vi "Camera.vi"(8 "error in (no error)":errorcluster, 10 "Notifiers":T1, 11 "All Message Queue Cluster":T2) -> (0 "error out":errorcluster)   [LabVIEW 2013]
doc: "Ce VI est la partie visualisation du Spectrometre. Elle permet l'envoie d'ordre à cette appareil et affiche son état.\n- Connected : indique si l'appareil est connecté.\n- Acquiring : indique si le spectrometre acquière.\n- Status : indique le status actuel du spectromètre. CAD s'il y a une erreur, ou s'il est en mouvement, etc ..."
uses:
  Lib QMH/AllMessageQueue Cluster.ctl
  Lib QMH/Message Cluster.ctl
  Lib Notifier/Notifier.ctl
  Camera UI data.ctl
  <vilib>/vision/Image Controls.llb/IMAQ Image.ctl
  Camera config.ctl
  Lib IHM Control/Front Panel Status.ctl
  support/Status.vi
  Lib QMH/MessageQueues.lvlib
  Lib IHM Control/IHM Control.lvlib
  Lib Notifier/Notifier.lvlib
panel:
  out "Acquiring":bool
  out "Status":string
  out "Connected":bool
  # "Camera"
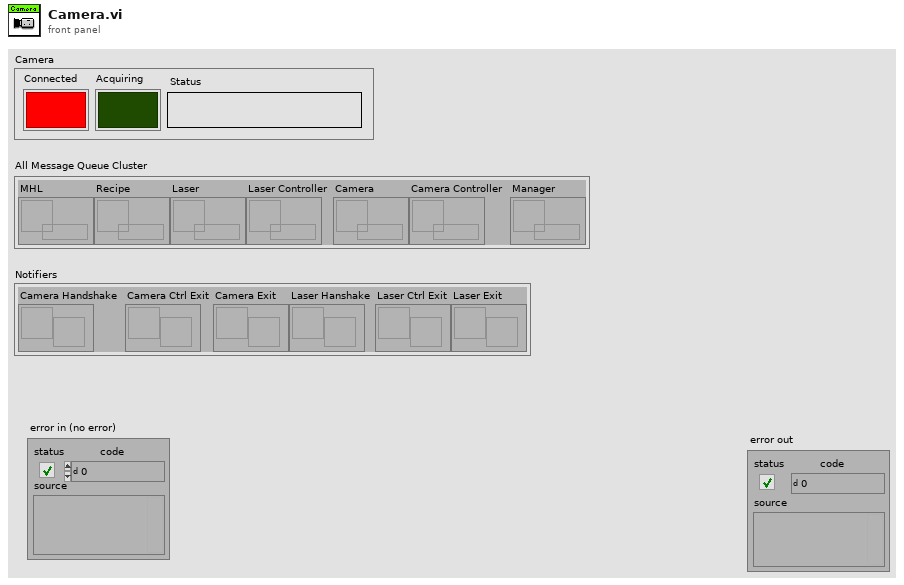
[diagram p1: front panel]
types:
  T1 = typedef "Notifier.lvlib/Notifier.ctl" = cluster{"Camera Handshake":refnum<notifier>, "Camera Ctrl Exit":refnum<notifier>, "Camera Exit":refnum<notifier>, "Laser Hanshake":refnum<notifier>, "Laser Ctrl Exit":refnum<notifier>, "Laser Exit":refnum<notifier>}
  T2 = typedef "MessageQueues.lvlib/AllMessageQueue Cluster.ctl" = cluster{"MHL":refnum<queue>, "Recipe":refnum<queue>, "Laser":refnum<queue>, "Laser Controller":refnum<queue>, "Camera":refnum<queue>, "Camera Controller":refnum<queue>, "Manager":refnum<queue>}
  T3 = typedef "IHM Control.lvlib/Front Panel Status.ctl" = enum16{"Initialisation", "Enable Laser", "Enable Camera", "Disable Laser", "Disable Camera"}
  T4 = typedef "Image Type" = u32
  T5 = typedef "Camera config.ctl" = cluster{"VISA resource name":refnum<visa-resource-name>}
  T6 = typedef "Camera UI data.ctl" = cluster{"Connected":bool, "Status":string, "Acquiring":bool, "Image":T7}
  T7 = typedef "IMAQ Image.ctl" = refnum<image>
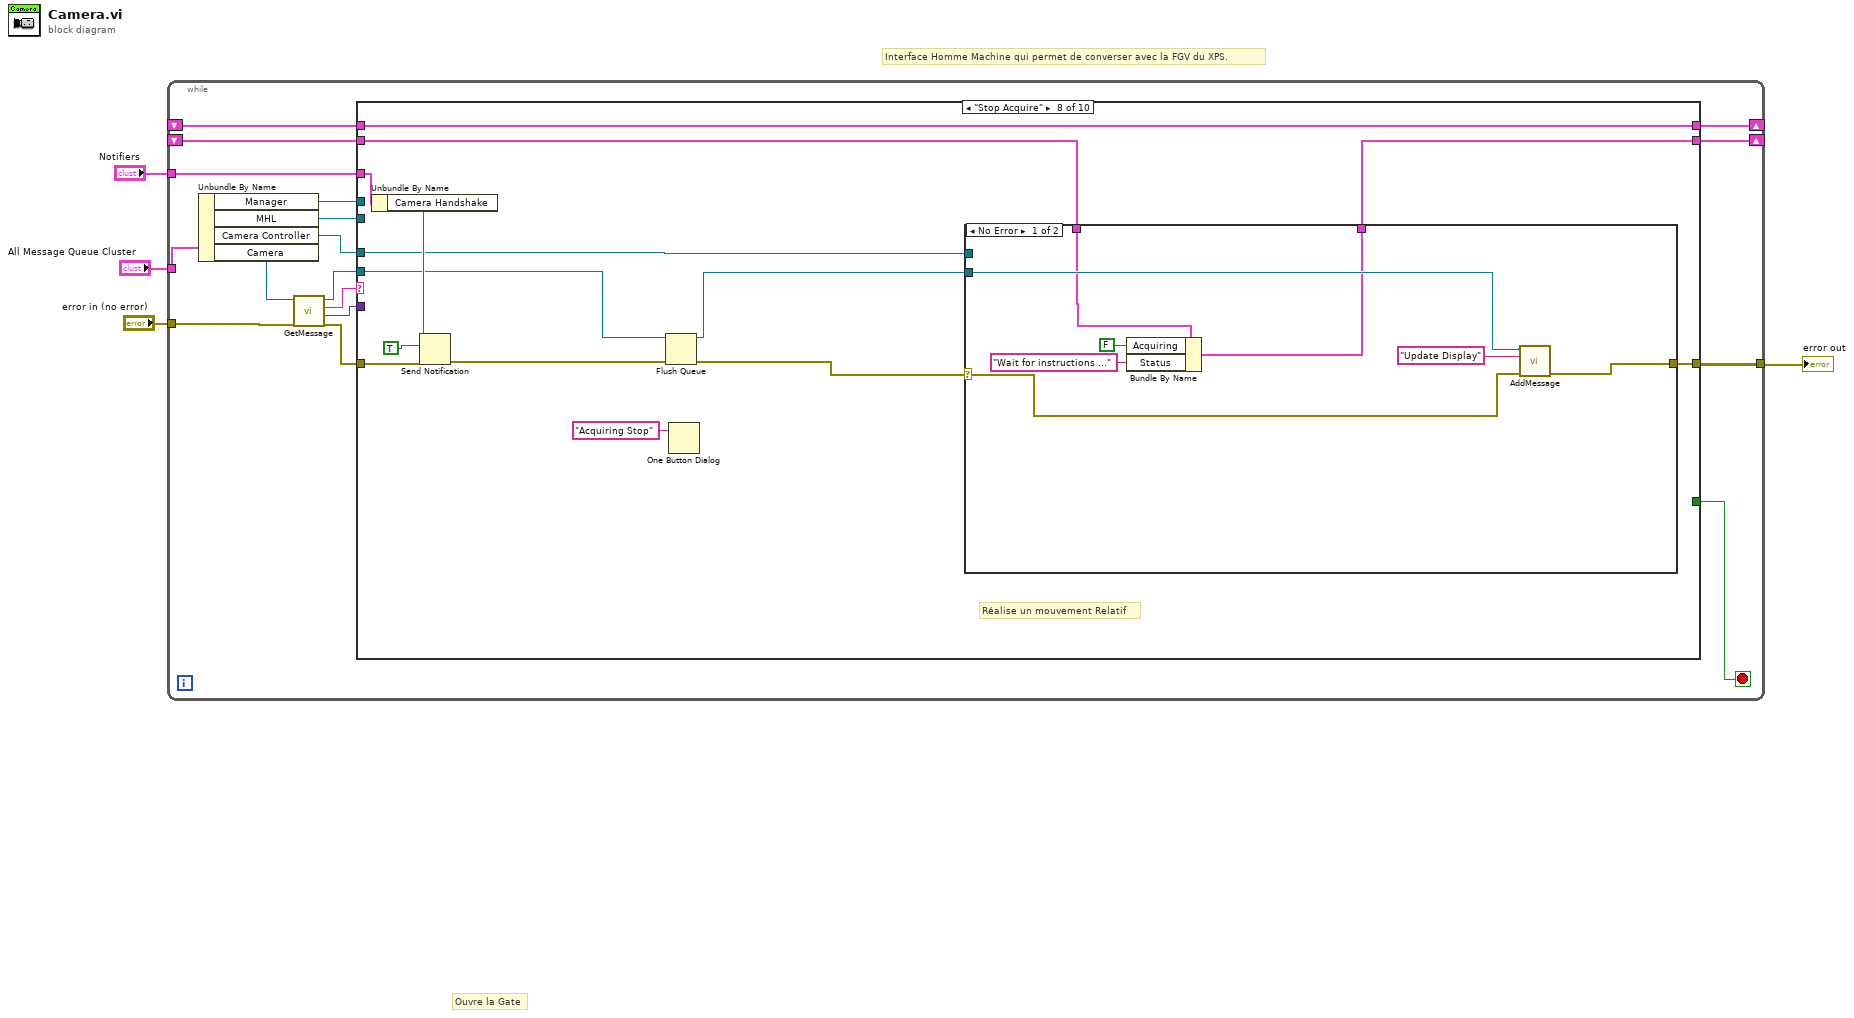
[diagram p0: block diagram]
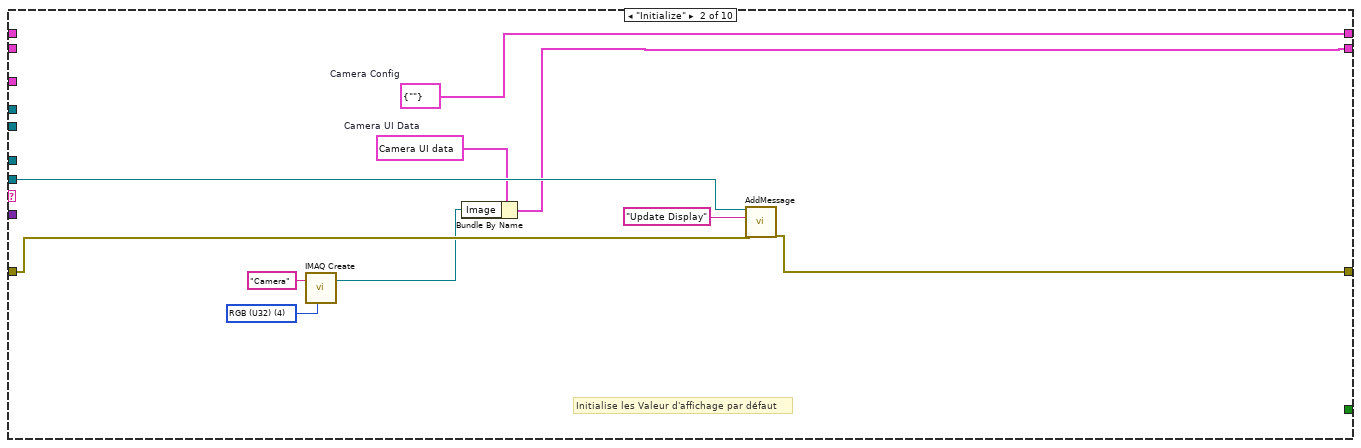
[diagram p3: hidden frame]
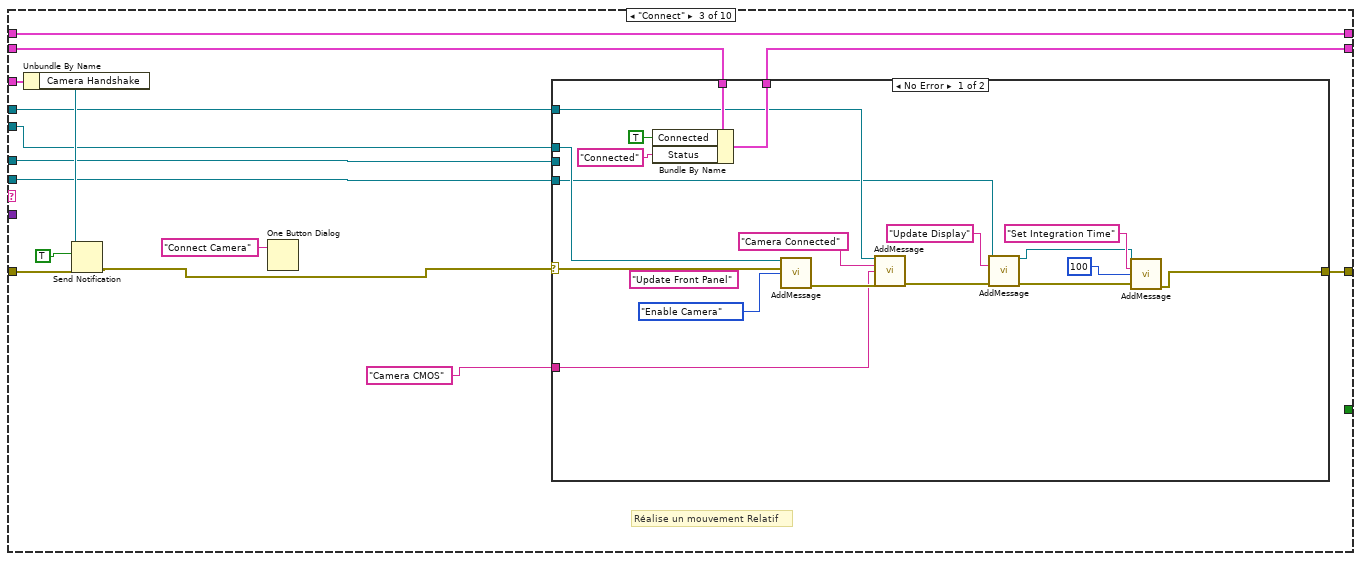
[diagram p4: hidden frame]
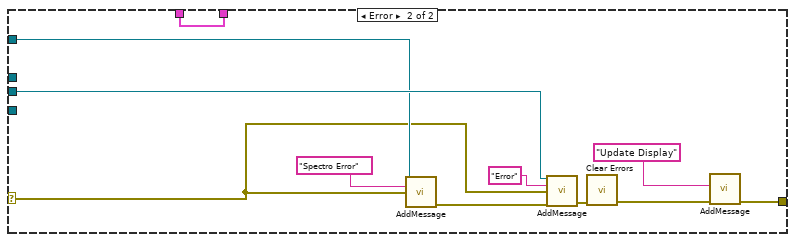
[diagram p5: hidden frame]
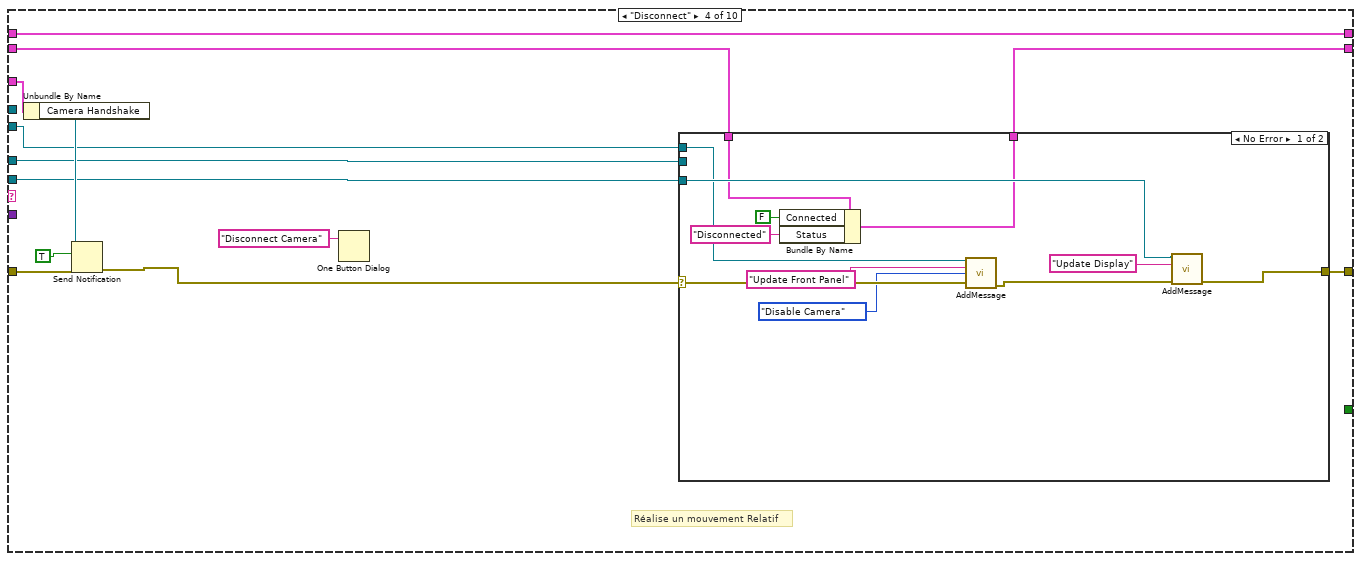
[diagram p6: hidden frame]
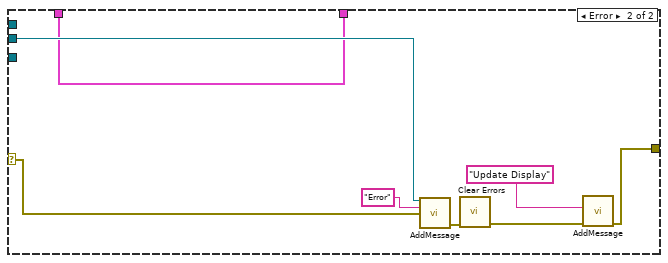
[diagram p7: hidden frame]
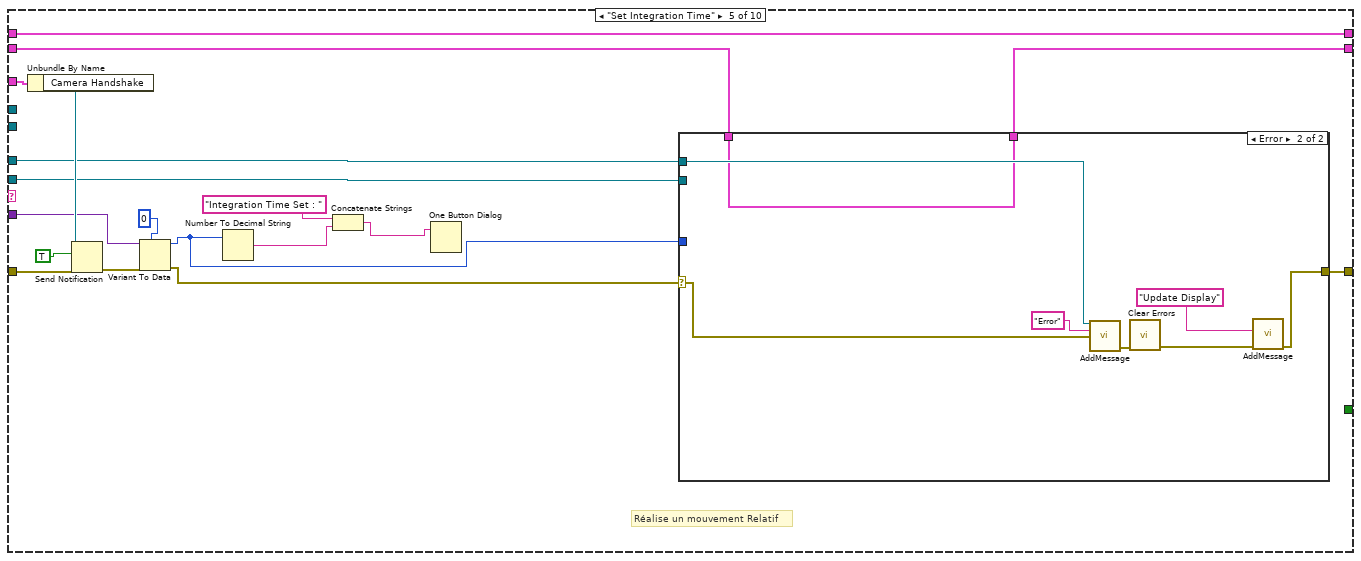
[diagram p8: hidden frame]
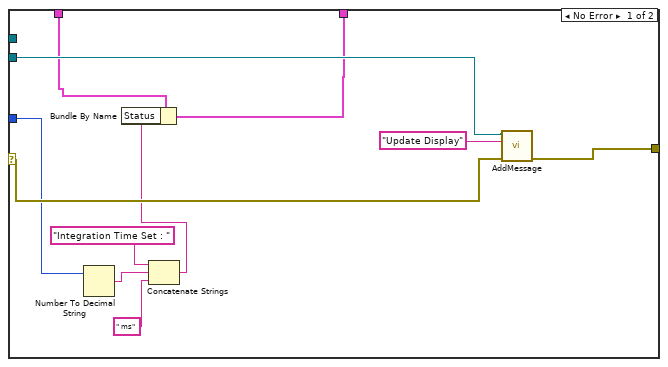
[diagram p9: hidden frame]
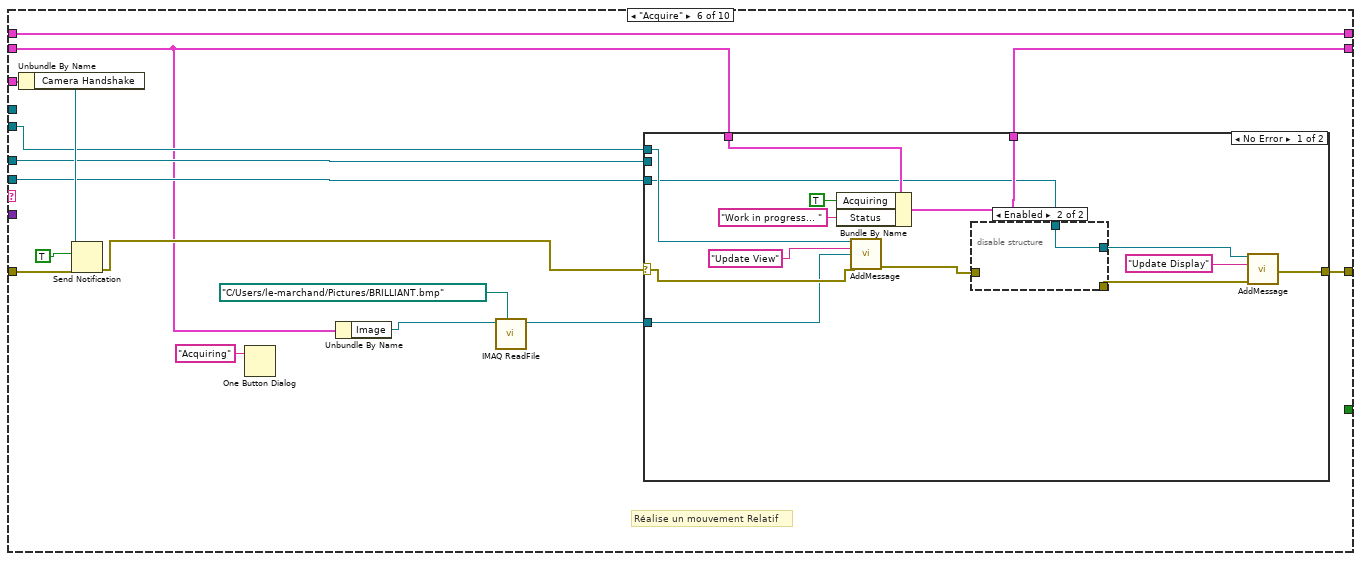
[diagram p10: hidden frame]
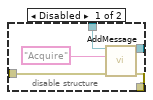
[diagram p11: hidden frame]
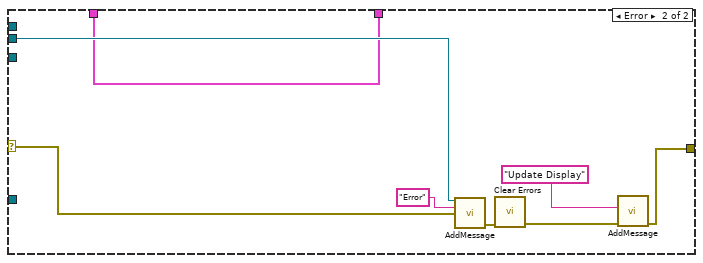
[diagram p12: hidden frame]
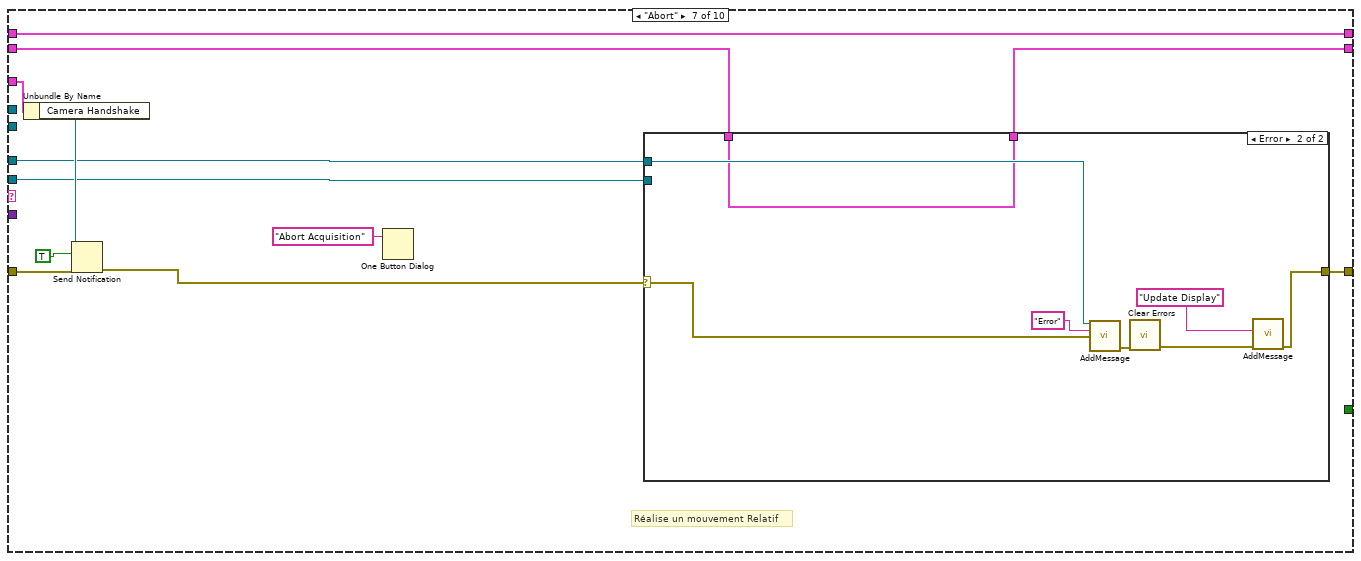
[diagram p13: hidden frame]
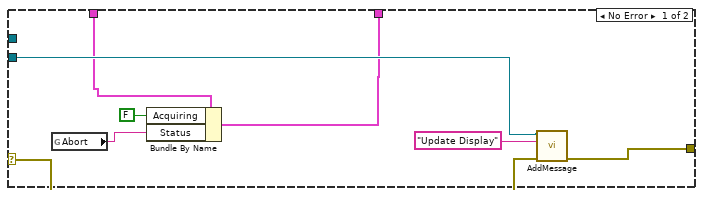
[diagram p14: hidden frame]
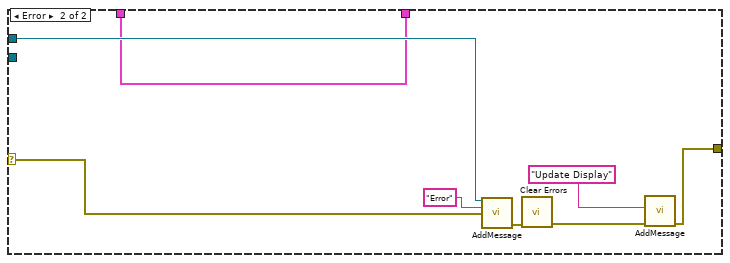
[diagram p15: hidden frame]
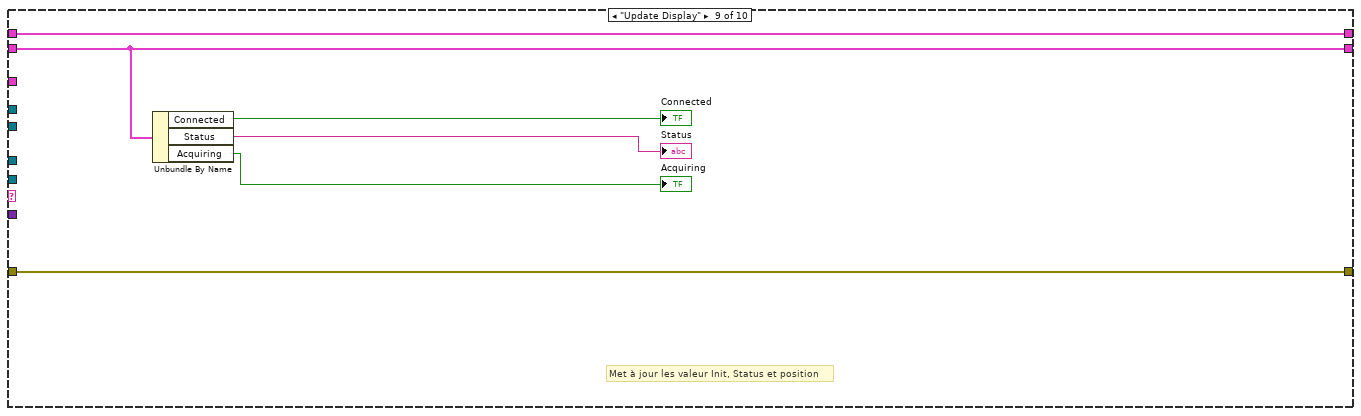
[diagram p16: hidden frame]
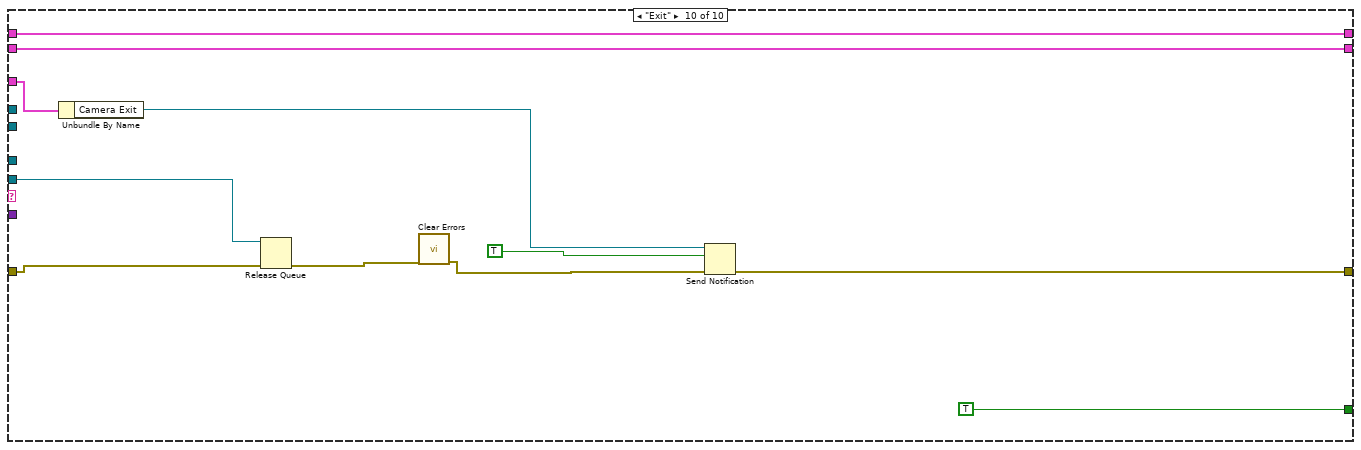
[diagram p17: hidden frame]
diagram:
  # "Interface Homme Machine qui permet de converser avec la FGV du XPS."
  # "Ouvre la Gate"
  n1 = while {
    tunnel: "All Message Queue Cluster" -> [w15]
    tunnel: "Notifiers" -> [w21]
    tunnel: "error in (no error)" -> [w16]
    tunnel: [w14] -> w1
    shift-right: [w10] -> _
    shift-left: _ -> [w11]
    shift-right: [w8] -> _
    shift-left: _ -> [w9]
    stop <- w12 stop-if-true
    n2 = Unbundle By Name(w15) -> ("Manager"=w5:refnum<queue>, "MHL"=w6:refnum<queue>, "Camera Controller"=w13:refnum<queue>, "Camera"=w7:refnum<queue>)
    n3 = call "GetMessage.vi"("entrée d'erreur"=w16, "Message queue"=w7) -> ("sortie d'erreur"=w17:errorcluster, "Data"=w18:variant, "Message"=w19:string, "Dup Message Queue"=w20:refnum<queue>)  [unwired: 6 in]
    n4 = case shown="\"Stop Acquire\"" w19 {
      tunnel: w21 -> [_ _ w47 w91 w129 w164 w204 w234 _ w268]
      tunnel: w20 -> [_ w31 w46 w90 w128 w163 w203 w225 _ w262]
      tunnel: w18 -> [_ _ _ _ w120 _ _ _ _ _]
      tunnel: w17 -> [w24 w33 w40 w84 w122 w158 w197 w228 w257 w263]
      tunnel: [w24 w32 w45 w89 w127 w162 w202 w233 w257 w265] -> w14
      tunnel: w13 -> [_ _ w44 w88 w126 w161 w201 w232 _ _]
      tunnel: [_ _ _ _ _ _ _ _ _ TRUE] -> w12
      tunnel: w11 -> [w23 _ w43 w87 w125 w160 w200 w231 w258 w264]
      tunnel: [w23 w30 w43 w87 w125 w160 w200 w231 w258 w264] -> w10
      tunnel: w9 -> [w22 _ w42 w86 w124 w152 w199 w230 w256 w261]
      tunnel: [w22 w28 w41 w85 w123 w159 w198 w229 w256 w261] -> w8
      tunnel: w6 -> [_ _ w39 w83 _ w157 _ _ _ _]
      tunnel: w5 -> [_ _ w38 _ _ _ _ _ _ _]
      frame Default {
        # "ne fait rien si le message dépilé n'existe pas"
      }
      frame "Initialize" {
        w26 = T4 4 items=["Grayscale (U8)", "Grayscale (I16)", "Grayscale (SGL)", "Complex (CSG)", "RGB (U32)", "HSL (U32)", "RGB (U64)", "Grayscale (U16)"] ("Image Type")
        w30 = T5 {"VISA resource name"=""}  # Camera Config
        w29 = T6 {"Connected"=FALSE, "Status"="", "Acquiring"=FALSE, "Image"=refnum}  # Camera UI Data
        # "Initialise les Valeur d'affichage par défaut"
        n5 = call "IMAQ Create"("Image Name"="Camera", "Image Type"=w26) -> ("New Image"=w25:T7)  [unwired: 3 in, 1 out]
        n6 = Bundle By Name(cluster=w29, "Image"=w25) -> (w28:T6)
        n7 = call "AddMessage.vi"("Message queue"=w31, "Message"="Update Display", "entrée d'erreur (pas d'erreur)"=w33) -> ("error out"=w32:errorcluster)  [unwired: 11 in, 1 out]
      }
      frame "Connect" {
        # "Réalise un mouvement Relatif"
        n8 = Unbundle By Name(w47) -> ("Camera Handshake"=w49:refnum<notifier>)
        n9 = Send Notification(notification=TRUE, notifier=w49, error in (no error)=w40) -> (error out=w35:errorcluster)  [unwired: 1 out]
        n10 = One Button Dialog(message="Connect Camera") -> ()  [unwired: 1 in, 1 out]
        n11 = case shown="No Error" w35 {
          selector: w35 -> [w65 w71]
          tunnel: w46 -> [w54 _]
          tunnel: [w55 w76] -> w45
          tunnel: w44 -> [_ w75]
          tunnel: w42 -> [w68 w74]
          tunnel: [w67 w74] -> w41
          tunnel: w39 -> [w59 _]
          tunnel: w38 -> [w62 w72]
          tunnel: "Camera CMOS" -> [w51 _]
          frame No Error {
            n12 = Bundle By Name(cluster=w68, "Connected"=TRUE, "Status"="Connected") -> (w67:T6)
            n13 = call "AddMessage.vi"("Message queue"=w59, "Message"="Update Front Panel", "Data"=Front_Panel_Status."Enable Camera" ("Front Panel status"), "entrée d'erreur (pas d'erreur)"=w65) -> ("error out"=w58:errorcluster)  [unwired: 10 in, 1 out]
            n14 = call "AddMessage.vi"("Message queue"=w62, "Message"="Camera Connected", "Data"=w51, "entrée d'erreur (pas d'erreur)"=w58) -> ("error out"=w57:errorcluster)  [unwired: 10 in, 1 out]
            n15 = call "AddMessage.vi"("Message queue"=w54, "Message"="Update Display", "entrée d'erreur (pas d'erreur)"=w57) -> ("Dup Message queue"=w50:refnum<queue>, "error out"=w56:errorcluster)  [unwired: 11 in]
            n16 = call "AddMessage.vi"("Message queue"=w50, "Message"="Set Integration Time", "Data"=100 ("index"), "entrée d'erreur (pas d'erreur)"=w56) -> ("error out"=w55:errorcluster)  [unwired: 10 in, 1 out]
          }
          frame Error {
            n17 = call "AddMessage.vi"("Message queue"=w72, "Message"="Spectro Error", "Data"=w71) -> ("error out"=w70:errorcluster)  [unwired: 11 in, 1 out]
            n18 = call "AddMessage.vi"("Message queue"=w75, "Message"="Error", "Data"=w71, "entrée d'erreur (pas d'erreur)"=w70) -> ("error out"=w79:errorcluster)  [unwired: 10 in, 1 out]
            n19 = call <vilib>:"Clear Errors.vi"("error in (no error)"=w79) -> ("error out"=w77:errorcluster)  [unwired: 6 in]
            n20 = call "AddMessage.vi"("Message"="Update Display", "entrée d'erreur (pas d'erreur)"=w77) -> ("error out"=w76:errorcluster)  [unwired: 12 in, 1 out]
          }
        }
      }
      frame "Disconnect" {
        # "Réalise un mouvement Relatif"
        n21 = Unbundle By Name(w91) -> ("Camera Handshake"=w93:refnum<notifier>)
        n22 = Send Notification(notification=TRUE, notifier=w93, error in (no error)=w84) -> (error out=w82:errorcluster)  [unwired: 1 out]
        n23 = One Button Dialog(message="Disconnect Camera") -> ()  [unwired: 1 in, 1 out]
        n24 = case shown="No Error" w82 {
          selector: w82 -> [w99 w108]
          tunnel: w90 -> [w105 _]
          tunnel: [w103 w109] -> w89
          tunnel: w88 -> [_ w107]
          tunnel: w86 -> [w102 w106]
          tunnel: [w101 w106] -> w85
          tunnel: w83 -> [w97 _]
          frame No Error {
            n25 = Bundle By Name(cluster=w102, "Connected"=FALSE, "Status"="Disconnected") -> (w101:T6)
            n26 = call "AddMessage.vi"("Message queue"=w97, "Message"="Update Front Panel", "Data"=Front_Panel_Status."Disable Camera" ("Front Panel status"), "entrée d'erreur (pas d'erreur)"=w99) -> ("error out"=w98:errorcluster)  [unwired: 10 in, 1 out]
            n27 = call "AddMessage.vi"("Message queue"=w105, "Message"="Update Display", "entrée d'erreur (pas d'erreur)"=w98) -> ("error out"=w103:errorcluster)  [unwired: 11 in, 1 out]
          }
          frame Error {
            n28 = call "AddMessage.vi"("Message queue"=w107, "Message"="Error", "Data"=w108) -> ("error out"=w112:errorcluster)  [unwired: 11 in, 1 out]
            n29 = call <vilib>:"Clear Errors.vi"("error in (no error)"=w112) -> ("error out"=w110:errorcluster)  [unwired: 6 in]
            n30 = call "AddMessage.vi"("Message"="Update Display", "entrée d'erreur (pas d'erreur)"=w110) -> ("error out"=w109:errorcluster)  [unwired: 12 in, 1 out]
          }
        }
      }
      frame "Set Integration Time" {
        # "Réalise un mouvement Relatif"
        n31 = Unbundle By Name(w129) -> ("Camera Handshake"=w131:refnum<notifier>)
        n32 = Send Notification(notification=TRUE, notifier=w131, error in (no error)=w122) -> (error out=w121:errorcluster)  [unwired: 1 out]
        n33 = Variant To Data(error in=w121, type=0, Variant=w120) -> (data=w114:i32, error out=w118:errorcluster)
        n34 = Number To Decimal String(number=w114) -> (decimal integer string=w117:string)  [unwired: 1 in]
        n35 = Concatenate Strings("Integration Time Set : " ("string"), w117) -> (w115:string)
        n36 = One Button Dialog(message=w115) -> ()  [unwired: 1 in, 1 out]
        n37 = case shown="Error" w118 {
          selector: w118 -> [w139 w145]
          tunnel: w128 -> [w142 _]
          tunnel: [w140 w146] -> w127
          tunnel: w126 -> [_ w144]
          tunnel: w124 -> [w138 w143]
          tunnel: [w137 w143] -> w123
          tunnel: w114 -> [w132 _]
          frame No Error {
            n38 = Number To Decimal String(number=w132) -> (decimal integer string=w135:string)  [unwired: 1 in]
            n39 = Concatenate Strings("Integration Time Set : " ("string"), w135, " ms" ("string")) -> (w133:string)
            n40 = Bundle By Name(cluster=w138, "Status"=w133) -> (w137:T6)
            n41 = call "AddMessage.vi"("Message queue"=w142, "Message"="Update Display", "entrée d'erreur (pas d'erreur)"=w139) -> ("error out"=w140:errorcluster)  [unwired: 11 in, 1 out]
          }
          frame Error {
            n42 = call "AddMessage.vi"("Message queue"=w144, "Message"="Error", "Data"=w145) -> ("error out"=w149:errorcluster)  [unwired: 11 in, 1 out]
            n43 = call <vilib>:"Clear Errors.vi"("error in (no error)"=w149) -> ("error out"=w147:errorcluster)  [unwired: 6 in]
            n44 = call "AddMessage.vi"("Message"="Update Display", "entrée d'erreur (pas d'erreur)"=w147) -> ("error out"=w146:errorcluster)  [unwired: 12 in, 1 out]
          }
        }
      }
      frame "Acquire" {
        # "Réalise un mouvement Relatif"
        n45 = Unbundle By Name(w164) -> ("Camera Handshake"=w166:refnum<notifier>)
        n46 = Send Notification(notification=TRUE, notifier=w166, error in (no error)=w158) -> (error out=w156:errorcluster)  [unwired: 1 out]
        n47 = One Button Dialog(message="Acquiring") -> ()  [unwired: 1 in, 1 out]
        n48 = Unbundle By Name(w152) -> ("Image"=w151:T7)
        n49 = call "IMAQ ReadFile"("File Path"=path "C:/Users/le-marchand/Pictures/BRILLIANT.bmp", "Image"=w151) -> ("Image Out"=w153:T7)  [unwired: 5 in, 4 out]
        n50 = case shown="No Error" w156 {
          selector: w156 -> [w172 w189]
          tunnel: w163 -> [w169 _]
          tunnel: [w179 w190] -> w162
          tunnel: w161 -> [_ w188]
          tunnel: w152 -> [w177 w187]
          tunnel: [w176 w187] -> w159
          tunnel: w157 -> [w173 _]
          tunnel: w153 -> [w168 _]
          frame No Error {
            n51 = Bundle By Name(cluster=w177, "Acquiring"=TRUE ("Connected"), "Status"="Work in progress... ") -> (w176:T6)
            n52 = call "AddMessage.vi"("Message queue"=w173, "Message"="Update View", "Data"=w168, "entrée d'erreur (pas d'erreur)"=w172) -> ("error out"=w171:errorcluster)  [unwired: 10 in, 1 out]
            n53 = disable-structure shown="Enabled" {
              disable-tunnel: w171 -> [w184 _]
              disable-tunnel: [w183 _] -> w170
              disable-tunnel: w169 -> [w182 w186]
              disable-tunnel: [w181 w186] -> w167
              frame Disabled {
                n54 = call "AddMessage.vi"("Message queue"=w182, "Message"="Acquire", "entrée d'erreur (pas d'erreur)"=w184) -> ("Dup Message queue"=w181:refnum<queue>, "error out"=w183:errorcluster)  [unwired: 11 in]
              }
              frame Enabled {
              }
            }
            n55 = call "AddMessage.vi"("Message queue"=w167, "Message"="Update Display", "entrée d'erreur (pas d'erreur)"=w170) -> ("error out"=w179:errorcluster)  [unwired: 11 in, 1 out]
          }
          frame Error {
            n56 = call "AddMessage.vi"("Message queue"=w188, "Message"="Error", "Data"=w189) -> ("error out"=w193:errorcluster)  [unwired: 11 in, 1 out]
            n57 = call <vilib>:"Clear Errors.vi"("error in (no error)"=w193) -> ("error out"=w191:errorcluster)  [unwired: 6 in]
            n58 = call "AddMessage.vi"("Message"="Update Display", "entrée d'erreur (pas d'erreur)"=w191) -> ("error out"=w190:errorcluster)  [unwired: 12 in, 1 out]
          }
        }
      }
      frame "Abort" {
        # "Réalise un mouvement Relatif"
        n59 = Unbundle By Name(w204) -> ("Camera Handshake"=w206:refnum<notifier>)
        n60 = Send Notification(notification=TRUE, notifier=w206, error in (no error)=w197) -> (error out=w196:errorcluster)  [unwired: 1 out]
        n61 = One Button Dialog(message="Abort Acquisition") -> ()  [unwired: 1 in, 1 out]
        n62 = case shown="Error" w196 {
          selector: w196 -> [w211 w217]
          tunnel: w203 -> [w214 _]
          tunnel: [w212 w218] -> w202
          tunnel: w201 -> [_ w216]
          tunnel: w199 -> [w209 w215]
          tunnel: [w208 w215] -> w198
          frame No Error {
            n63 = global read "Status.vi" "Abort"() -> (w207:string)
            n64 = Bundle By Name(cluster=w209, "Acquiring"=FALSE ("Connected"), "Status"=w207) -> (w208:T6)
            n65 = call "AddMessage.vi"("Message queue"=w214, "Message"="Update Display", "entrée d'erreur (pas d'erreur)"=w211) -> ("error out"=w212:errorcluster)  [unwired: 11 in, 1 out]
          }
          frame Error {
            n66 = call "AddMessage.vi"("Message queue"=w216, "Message"="Error", "Data"=w217) -> ("error out"=w221:errorcluster)  [unwired: 11 in, 1 out]
            n67 = call <vilib>:"Clear Errors.vi"("error in (no error)"=w221) -> ("error out"=w219:errorcluster)  [unwired: 6 in]
            n68 = call "AddMessage.vi"("Message"="Update Display", "entrée d'erreur (pas d'erreur)"=w219) -> ("error out"=w218:errorcluster)  [unwired: 12 in, 1 out]
          }
        }
      }
      frame "Stop Acquire" {
        # "Réalise un mouvement Relatif"
        n69 = Unbundle By Name(w234) -> ("Camera Handshake"=w236:refnum<notifier>)
        n70 = Send Notification(notification=TRUE, notifier=w236, error in (no error)=w228) -> (error out=w227:errorcluster)  [unwired: 1 out]
        n71 = Flush Queue(queue=w225, error in (no error)=w227) -> (queue out=w224:refnum<queue>, error out=w226:errorcluster)  [unwired: 1 out]
        n72 = One Button Dialog(message="Acquiring Stop") -> ()  [unwired: 1 in, 1 out]
        n73 = case shown="No Error" w226 {
          selector: w226 -> [w241 w247]
          tunnel: w224 -> [w244 _]
          tunnel: [w242 w248] -> w233
          tunnel: w232 -> [_ w246]
          tunnel: w230 -> [w239 w245]
          tunnel: [w238 w245] -> w229
          frame No Error {
            n74 = Bundle By Name(cluster=w239, "Acquiring"=FALSE ("Connected"), "Status"="Wait for instructions ...") -> (w238:T6)
            n75 = call "AddMessage.vi"("Message queue"=w244, "Message"="Update Display", "entrée d'erreur (pas d'erreur)"=w241) -> ("error out"=w242:errorcluster)  [unwired: 11 in, 1 out]
          }
          frame Error {
            n76 = call "AddMessage.vi"("Message queue"=w246, "Message"="Error", "Data"=w247) -> ("error out"=w251:errorcluster)  [unwired: 11 in, 1 out]
            n77 = call <vilib>:"Clear Errors.vi"("error in (no error)"=w251) -> ("error out"=w249:errorcluster)  [unwired: 6 in]
            n78 = call "AddMessage.vi"("Message"="Update Display", "entrée d'erreur (pas d'erreur)"=w249) -> ("error out"=w248:errorcluster)  [unwired: 12 in, 1 out]
          }
        }
      }
      frame "Update Display" {
        # "Met à jour les valeur Init, Status et position"
        n79 = Unbundle By Name(w256) -> ("Connected"=→"Connected":bool, "Status"=→"Status":string, "Acquiring"=→"Acquiring":bool)
      }
      frame "Exit" {
        n80 = Unbundle By Name(w268) -> ("Camera Exit"=w267:refnum<notifier>)
        n81 = Release Queue(queue=w262, error in (no error)=w263) -> (error out=w259:errorcluster)  [unwired: 1 in, 2 out]
        n82 = call <vilib>:"Clear Errors.vi"("error in (no error)"=w259) -> ("error out"=w260:errorcluster)  [unwired: 6 in]
        n83 = Send Notification(notification=TRUE, notifier=w267, error in (no error)=w260) -> (error out=w265:errorcluster)  [unwired: 1 out]
      }
    }
  }
  "error out" <- w1
